vi "GETVelocity.vi"(8 "error in (no error)":errorcluster, 11 "Tapedrive_ESP301 in":refnum<class "Tapedrive_ESP301.lvclass">) -> (0 "error out":errorcluster, 3 "Tapedrive_ESP301 out":refnum<class "Tapedrive_ESP301.lvclass">)   [LabVIEW 2013, in "Tapedrive_ESP301.lvclass"]
uses:
  Tapedrive_ESP301.lvclass
panel:
  out "Array 2":dbl[](array[numeric])
  out "Array":bool[](array[boolean])
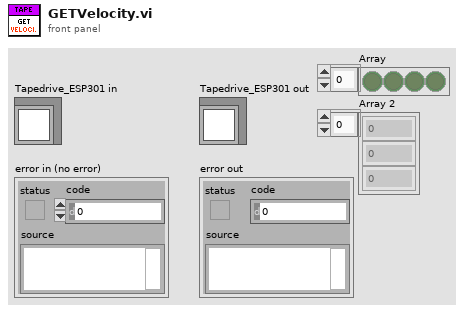
[diagram p1: front panel]
types:
  T1 = cluster{"Axis 1":cluster{"Value":dbl, "Min":dbl, "Max":dbl, "StepSize":dbl, "Tolerance":dbl, "ValueActual":dbl}, "Axis 2":cluster{"Value":dbl, "Min":dbl, "Max":dbl, "StepSize":dbl, "Tolerance":dbl, "ValueActual":dbl}}
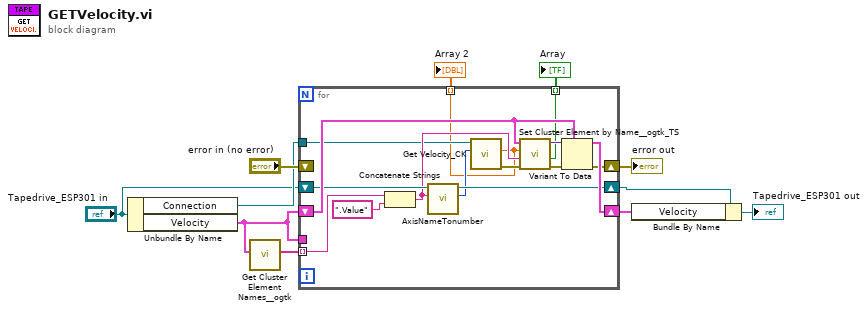
[diagram p0: block diagram]
diagram:
  n1 = Unbundle By Name("Tapedrive_ESP301 in") -> ("Connection"=w7:refnum<visa-resource-name>, "Velocity"=w3:T1)
  n2 = call <userlib>:"Get Cluster Element Names__ogtk.vi"("Cluster"=w3) -> ("Element Names"=w4:string[])  [unwired: 9 in, 1 out]
  n3 = for {
    tunnel: w4 -> [w18] mode=indexing
    tunnel: w3 -> [_]
    shift-right: [w22] -> w5
    shift-left: w3 -> [w23]
    shift-right: [w20] -> w10
    shift-left: "Tapedrive_ESP301 in" -> [w21]
    tunnel: w7 -> [w14]
    shift-right: [w19] -> w9
    shift-left: "error in (no error)" -> [_]
    tunnel: [w13] -> w2 mode=indexing
    tunnel: [w12] -> w1 mode=indexing
    n4 = Concatenate Strings(w18, ".Value" ("string")) -> (w17:string)
    n5 = call "AxisNameTonumber.vi"("Channel"=w17, "Tapedrive_ESP301 in"=w21) -> ("Axis No."=w16:i16, "Tapedrive_ESP301 out"=w20:refnum<class "Tapedrive_ESP301.lvclass">)  [unwired: 8 in]
    n6 = call "Get Velocity_CK.vi"("Axis (1)"=w16, "VISA resource name"=w14) -> ("error out"=w15:errorcluster, "Velocity (units/s)"=w12:dbl)  [unwired: 3 in, 1 out]
    n7 = call "Set Cluster Element by Name__ogtk_TS.vi"("error in (no error)"=w15, "Element Name (\"\": New Element Data Name)"=w17, "New Element Value"=w12, "Cluster"=w23) -> ("error out"=w25:errorcluster, "found?"=w13:bool, "VCluster out"=w24:variant)  [unwired: 5 in]
    n8 = Variant To Data(error in=w25, type=w23, Variant=w24) -> (data=w22:T1, error out=w19:errorcluster)
  }
  "error out" <- w9
  "Array" <- w2
  "Array 2" <- w1
  n9 = Bundle By Name(cluster=w10, "Velocity"=w5) -> (→"Tapedrive_ESP301 out":refnum<class "Tapedrive_ESP301.lvclass">)
